vi "Force Close Log File Instance.vi"(8 "error in (no error)":errorcluster, 11 "Triggered Log in":refnum<class "Triggered Log.lvclass">) -> (0 "error out":errorcluster, 3 "Triggered Log out":refnum<class "Triggered Log.lvclass">)   [LabVIEW 2015, in "Triggered Log.lvclass"]
doc: "Flushes any data in the buffer and closes the current file instance. If the segmented log has reached its maximum limit for file instances, then the triggered log changes its state to complete and notifies any listeners that the state has changed."
uses:
  Triggered Log.lvclass
  Engine/Classes/Logs/Segmented Logs/Segmented Log/Segmented Log.lvclass
  Triggered Log State.ctl
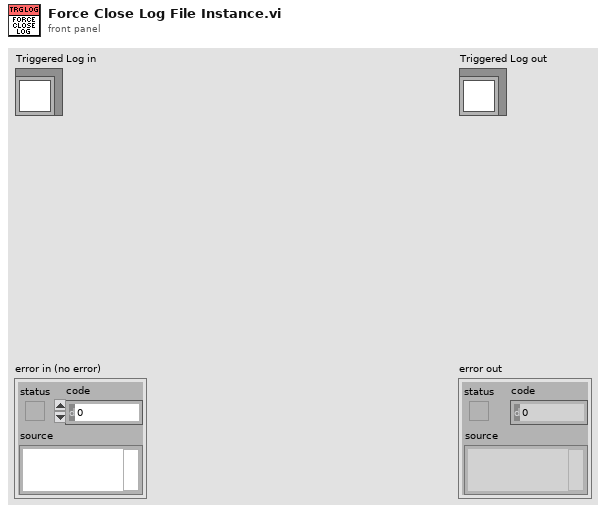
[diagram p1: front panel]
types:
  T1 = typedef "Triggered Log.lvclass/Triggered Log State.ctl" = enum16{"Waiting on Trigger", "Triggered", "Posttrigger", "Complete", "Idle", "Error"}
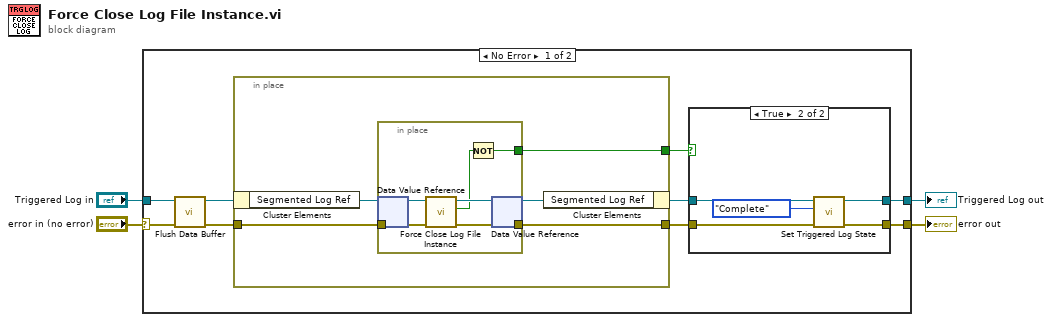
[diagram p0: block diagram]
diagram:
  n1 = case shown="No Error" "error in (no error)" {
    selector: "error in (no error)" -> [w13 w33]
    tunnel: [w6 w33] -> w3
    tunnel: [w7 w32] -> w1
    tunnel: "Triggered Log in" -> [w12 w32]
    frame No Error {
      n2 = call "Flush Data Buffer.vi"("error in (no error)"=w13, "Triggered Log in"=w12) -> ("error out"=w10:errorcluster, "Triggered Log out"=w11:refnum<class "Triggered Log.lvclass">)  [unwired: 8 in]
      n3 = in-place {
        in-place-border: w10 -> [w23]
        in-place-border: [w22] -> w9
        in-place-border: [w21] -> w5
        n4 = in-place-cluster #1(w11) -> ("Segmented Log Ref"=w25:refnum<data-value>)
        n5 = in-place {
          in-place-border: w23 -> [w29]
          in-place-border: [w28] -> w22
          in-place-border: [w26] -> w21
          n6 = in-place-dvr #2(w25) -> (w31:refnum<class "Segmented Log.lvclass">)  [unwired: 1 out]
          n7 = call "Force Close Log File Instance.vi"("error in (no error)"=w29, "Segmented Log in"=w31) -> ("error out"=w28:errorcluster, "Log Active"=w27:bool, "Segmented Log out"=w30:refnum<class "Segmented Log.lvclass">)  [unwired: 7 in]
          n8 = Not(x=w27) -> (.not. x?=w26:bool)
          n9 = in-place-dvr #2(w30) -> (w24:refnum<data-value>)  [unwired: 1 out]
        }
        n10 = in-place-cluster #1("Segmented Log Ref"=w24) -> (w8:refnum<class "Triggered Log.lvclass">)
      }
      n11 = case shown="True" w5 {
        tunnel: w9 -> [w14 w20]
        tunnel: [w14 w19] -> w6
        tunnel: [w15 w18] -> w7
        tunnel: w8 -> [w15 w17]
        frame False {
        }
        frame True {
          n12 = call "Set Triggered Log State.vi"("error in (no error)"=w20, "Triggered Log State"=Triggered_Log_State."Complete", "Triggered Log in"=w17) -> ("error out"=w19:errorcluster, "Triggered Log out"=w18:refnum<class "Triggered Log.lvclass">)  [unwired: 7 in]
        }
      }
    }
    frame Error {
    }
  }
  "error out" <- w3
  "Triggered Log out" <- w1
